vi "Get Datalogger Enqueuer.vi"(8 "error in (no error)":errorcluster, 11 "Sensor in":refnum<class "Sensor.lvclass">) -> (0 "error out":errorcluster, 2 "Datalogger Enqueuer":refnum<class "Message Enqueuer.lvclass">, 3 "Sensor out":refnum<class "Sensor.lvclass">)   [LabVIEW 2018, in "Sensor.lvlib" / "Sensor.lvclass"]
uses:
  Sensor.lvclass
  <vilib>/ActorFramework/Message Enqueuer/Message Enqueuer.lvclass
  Sensor.lvclass/Sensor.ctl
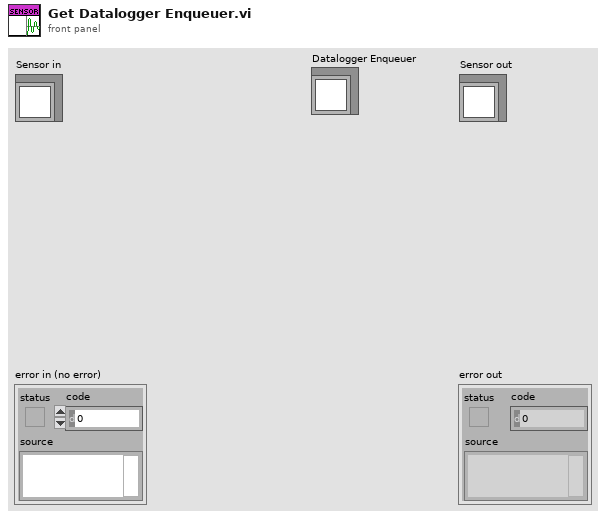
[diagram p1: front panel]
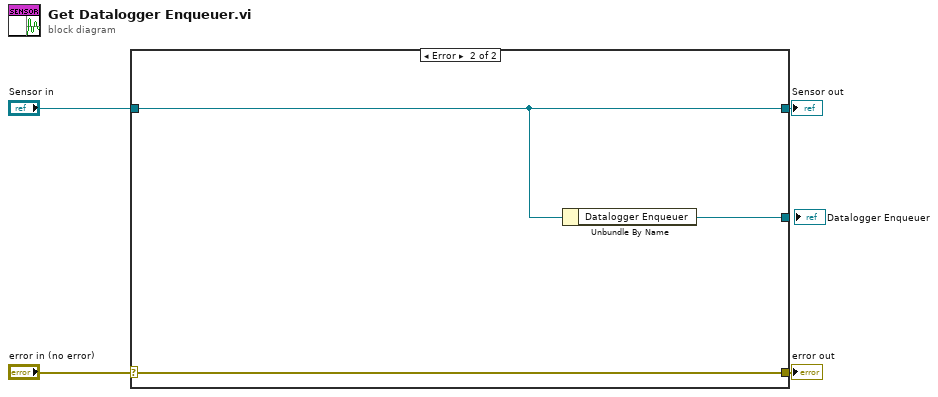
[diagram p0: block diagram]
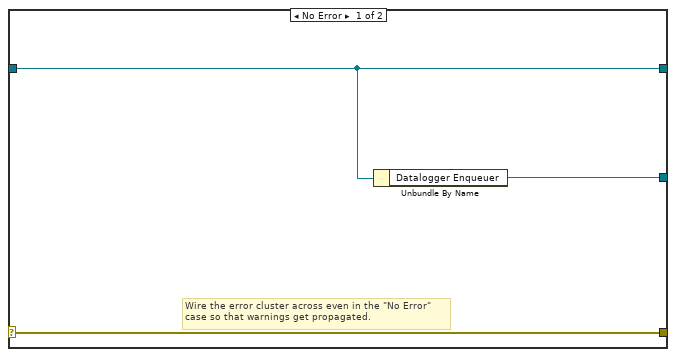
[diagram p2: hidden frame]
diagram:
  n1 = case shown="Error" "error in (no error)" {
    selector: "error in (no error)" -> [w7 w10]
    tunnel: [w7 w10] -> w3
    tunnel: [w5 w9] -> w1
    tunnel: "Sensor in" -> [w5 w9]
    tunnel: [w6 w8] -> _
    frame No Error {
      # "Wire the error cluster across even in the \"No Error\"\ncase so that warnings get propagated."
      n2 = Unbundle By Name(w5) -> ("Datalogger Enqueuer"=w6:refnum<class "Message Enqueuer.lvclass">)
    }
    frame Error {
      n3 = Unbundle By Name(w9) -> ("Datalogger Enqueuer"=w8:refnum<class "Message Enqueuer.lvclass">)
    }
  }
  "error out" <- w3
  "Sensor out" <- w1
